vi "Real Lorentzian Function.vi"(3 "output control":T1, 4 "data":variant, 5 "X":dbl[](array[numeric]), 6 "a":dbl[](array[numeric])) -> (0 "Error Out":errorcluster, 1 "f'(X,a)":dbl[][](array[numeric]), 2 "f(X,a)":dbl[](array[numeric]))   [LabVIEW 2016]
doc: "Sum of three Gaussians, plus DC offset."
uses:
  <vilib>/gmath/NumericalOptimization/LM_output select.ctl
  <vilib>/gmath/NI_Gmath.lvlib
panel:
  in  "Error In":errorcluster
  out "Waveform Graph":dbl[](graph)
  # "F0\nG\nA"
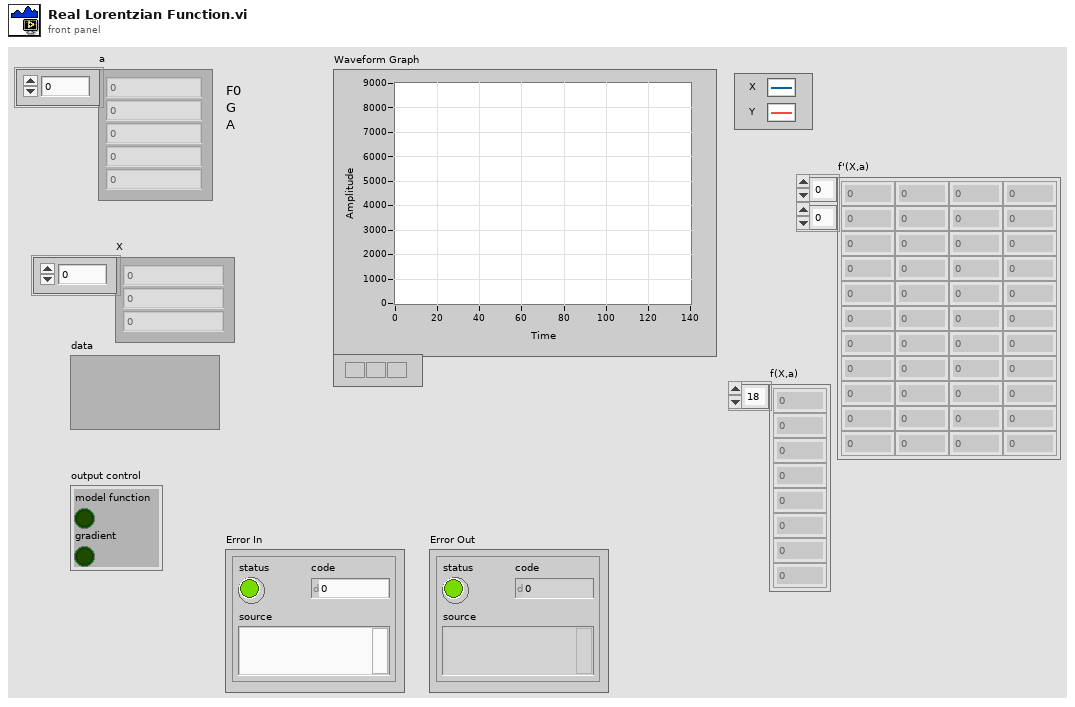
[diagram p1: front panel]
types:
  T1 = typedef "NI_Gmath.lvlib/LM_output select.ctl" = cluster{"model function":bool, "gradient":bool}
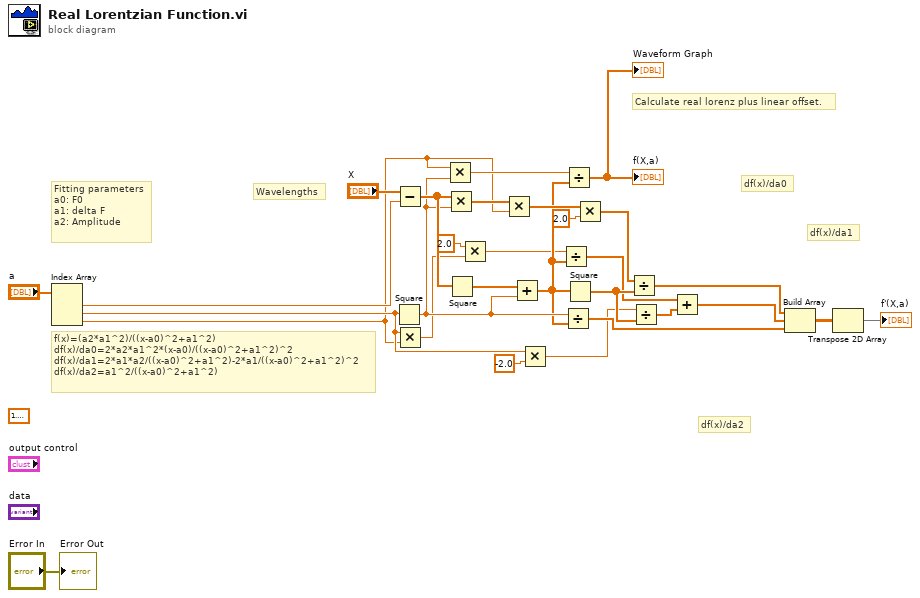
[diagram p0: block diagram]
diagram:
  (unwired) 1.5707963267948966
  # "df(x)/da0"
  # "df(x)/da1"
  # "df(x)/da2"
  # "Fitting parameters\na0: F0\na1: delta F\na2: Amplitude"
  # "Wavelengths"
  # "f(x)=(a2*a1^2)/((x-a0)^2+a1^2)\ndf(x)/da0=2*a2*a1^2*(x-a0)/((x-a0)^2+a1^2)^2\ndf(x)/da1=2*a1*a2/((x-a0)^2+a1^2)-2*a1/((x-a0)^2+a1^2)^2\ndf(x)/da2=a1^2/((x-a0)^2+a1^2)"
  # "Calculate real lorenz plus linear offset."
  n1 = Index Array(array="a") -> (element #1=w28:dbl, element #2=w11:dbl, element #3=w10:dbl)  [unwired: 3 in]
  n2 = Square(x=w11) -> (x^2=w19:dbl)
  n3 = Subtract(x="X", y=w28) -> (x-y=w20:dbl[])
  n4 = Multiply(x=w11, y=w10) -> (x*y=w9:dbl)
  n5 = Multiply(x=w10, y=w19) -> (x*y=w25:dbl)
  n6 = Multiply(x=w20, y=w19) -> (x*y=w18:dbl[])
  n7 = Square(x=w20) -> (x^2=w26:dbl[])
  n8 = Multiply(x=2.0, y=w9) -> (x*y=w7:dbl)
  n9 = Multiply(x=w18, y=w10) -> (x*y=w17:dbl[])
  n10 = Add(x=w26, y=w19) -> (x+y=w12:dbl[])
  n11 = Multiply(x=w11, y=-2.0) -> (x*y=w13:dbl)
  n12 = Divide(x=w7, y=w12) -> (x/y=w6:dbl[])
  n13 = Divide(x=w19, y=w12) -> (x/y=w23:dbl[])
  n14 = Divide(x=w25, y=w12) -> (x/y=→"f(X,a)" →"Waveform Graph":dbl[])
  n15 = Square(x=w12) -> (x^2=w15:dbl[])
  n16 = Multiply(x=w17, y=2.0) -> (x*y=w16:dbl[])
  n17 = Divide(x=w16, y=w15) -> (x/y=w22:dbl[])
  n18 = Divide(x=w13, y=w15) -> (x/y=w5:dbl[])
  n19 = Add(x=w6, y=w5) -> (x+y=w3:dbl[])
  n20 = Build Array(w22, w3, w23) -> (w2:dbl[][])
  n21 = Transpose 2D Array(2D array=w2) -> (transposed array=→"f'(X,a)":dbl[][])
  "Error Out" <- "Error In"
